vi "Read Discrete Inputs.vi"(8 "error in (no error)":errorcluster, 9 "number of discrete inputs":u16, 10 "starting address":u16, 11 "Modbus slave in":refnum<class "Modbus Slave.lvclass">) -> (0 "error out":errorcluster, 2 "discrete input values":bool[](array[boolean]), 3 "Modbus slave out":refnum<class "Modbus Slave.lvclass">)   [LabVIEW 2015, in "Modbus Slave.lvclass"]
doc: "Reads values of contiguous discrete inputs."
uses:
  <vilib>/Modbus/slave/Modbus Slave.lvclass
  <vilib>/Modbus/slave/Modbus Slave.lvclass/Modbus Slave.ctl
  <vilib>/Modbus/subvis/Data and Functions/Device Data Model/Device Data Model.lvclass
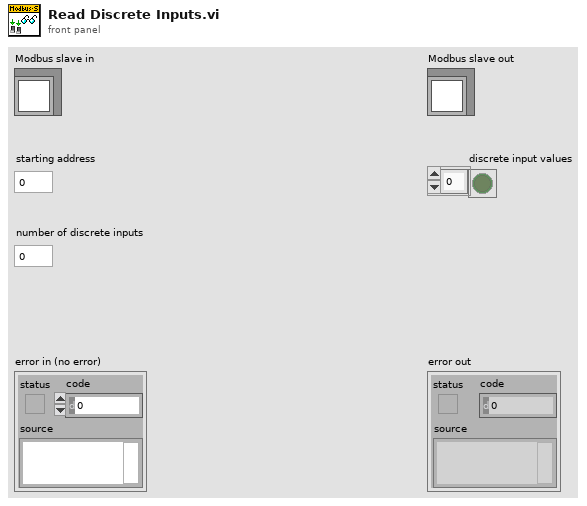
[diagram p1: front panel]
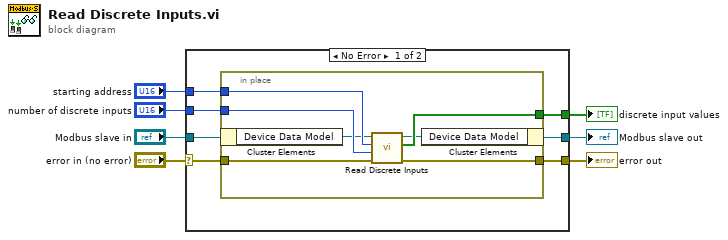
[diagram p0: block diagram]
diagram:
  n1 = case shown="No Error" "error in (no error)" {
    selector: "error in (no error)" -> [w8 w22]
    tunnel: "Modbus slave in" -> [w14 w23]
    tunnel: [w13 w23] -> w6
    tunnel: [w12 _] -> w5
    tunnel: "number of discrete inputs" -> [w11 _]
    tunnel: "starting address" -> [w10 _]
    tunnel: [w9 w22] -> w2
    frame No Error {
      n2 = in-place {
        in-place-border: [w21] -> w12
        in-place-border: w11 -> [w20]
        in-place-border: w10 -> [w19]
        in-place-border: [w18] -> w9
        in-place-border: w8 -> [w17]
        n3 = in-place-cluster #1(w14) -> ("Device Data Model"=w15:refnum<class "Device Data Model.lvclass">)
        n4 = call-dynamic "Read Discrete Inputs.vi"("error in (no error)"=w17, "number of inputs"=w20, "starting address"=w19, "device data model in"=w15) -> ("error out"=w18:errorcluster, "data"=w21:bool[], "device data model out"=w16:refnum<class "Device Data Model.lvclass">)  [unwired: 5 in]
        n5 = in-place-cluster #1("Device Data Model"=w16) -> (w13:refnum<class "Modbus Slave.lvclass">)
      }
    }
    frame Error {
    }
  }
  "error out" <- w2
  "Modbus slave out" <- w6
  "discrete input values" <- w5
